vi "SavePodDataToFile.vi"(10 "Configuration Data":T1, 11 "Config file Refnum in":T2) -> (3 "Config file Refnum out":T2)   [LabVIEW 2014]
uses:
  <vilib>/Utility/config.llb/Config Data RefNum.ctl
  <vilib>/Utility/config.llb/Write Key (I32).vi
  <vilib>/Utility/config.llb/Write Key (String).vi
  <vilib>/Utility/config.llb/Write Key (Double).vi
  <vilib>/Utility/config.llb/Write Key (Boolean).vi
  <vilib>/Utility/config.llb/NI_LVConfig.lvlib
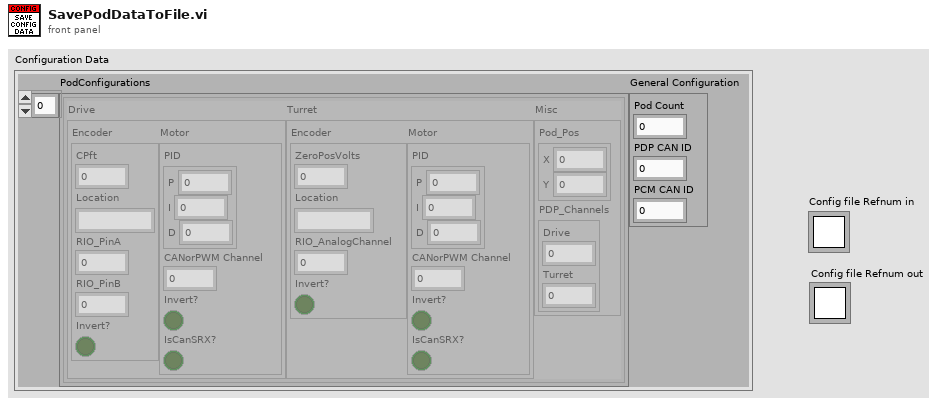
[diagram p1: front panel]
types:
  T1 = cluster{"PodConfigurations":cluster{"Drive":cluster{"Encoder":cluster{"CPft":dbl, "Location":string, "RIO_PinA":i32, "RIO_PinB":i32, "Invert?":bool}, "Motor":cluster{"PID":cluster{"P":dbl, "I":dbl, "D":dbl}, "CANorPWM Channel":i32, "Invert?":bool, "IsCanSRX?":bool}}, "Turret":cluster{"Encoder":cluster{"ZeroPosVolts":dbl, "Location":string, "RIO_AnalogChannel":i32, "Invert?":bool}, "Motor":cluster{"PID":cluster{"P":dbl, "I":dbl, "D":dbl}, "CANorPWM Channel":i32, "Invert?":bool, "IsCanSRX?":bool}}, "Misc":cluster{"Pod_Pos":cluster{"X":dbl, "Y":dbl}, "PDP_Channels":cluster{"Drive":i32, "Turret":i32}}}[], "General Configuration":cluster{"Pod Count":i32, "PDP CAN ID":i32, "PCM CAN ID":i32}}
  T2 = typedef "NI_LVConfig.lvlib/Config Data RefNum.ctl" = refnum<k1>
  T3 = cluster{"Drive":cluster{"Encoder":cluster{"CPft":dbl, "Location":string, "RIO_PinA":i32, "RIO_PinB":i32, "Invert?":bool}, "Motor":cluster{"PID":cluster{"P":dbl, "I":dbl, "D":dbl}, "CANorPWM Channel":i32, "Invert?":bool, "IsCanSRX?":bool}}, "Turret":cluster{"Encoder":cluster{"ZeroPosVolts":dbl, "Location":string, "RIO_AnalogChannel":i32, "Invert?":bool}, "Motor":cluster{"PID":cluster{"P":dbl, "I":dbl, "D":dbl}, "CANorPWM Channel":i32, "Invert?":bool, "IsCanSRX?":bool}}, "Misc":cluster{"Pod_Pos":cluster{"X":dbl, "Y":dbl}, "PDP_Channels":cluster{"Drive":i32, "Turret":i32}}}[]
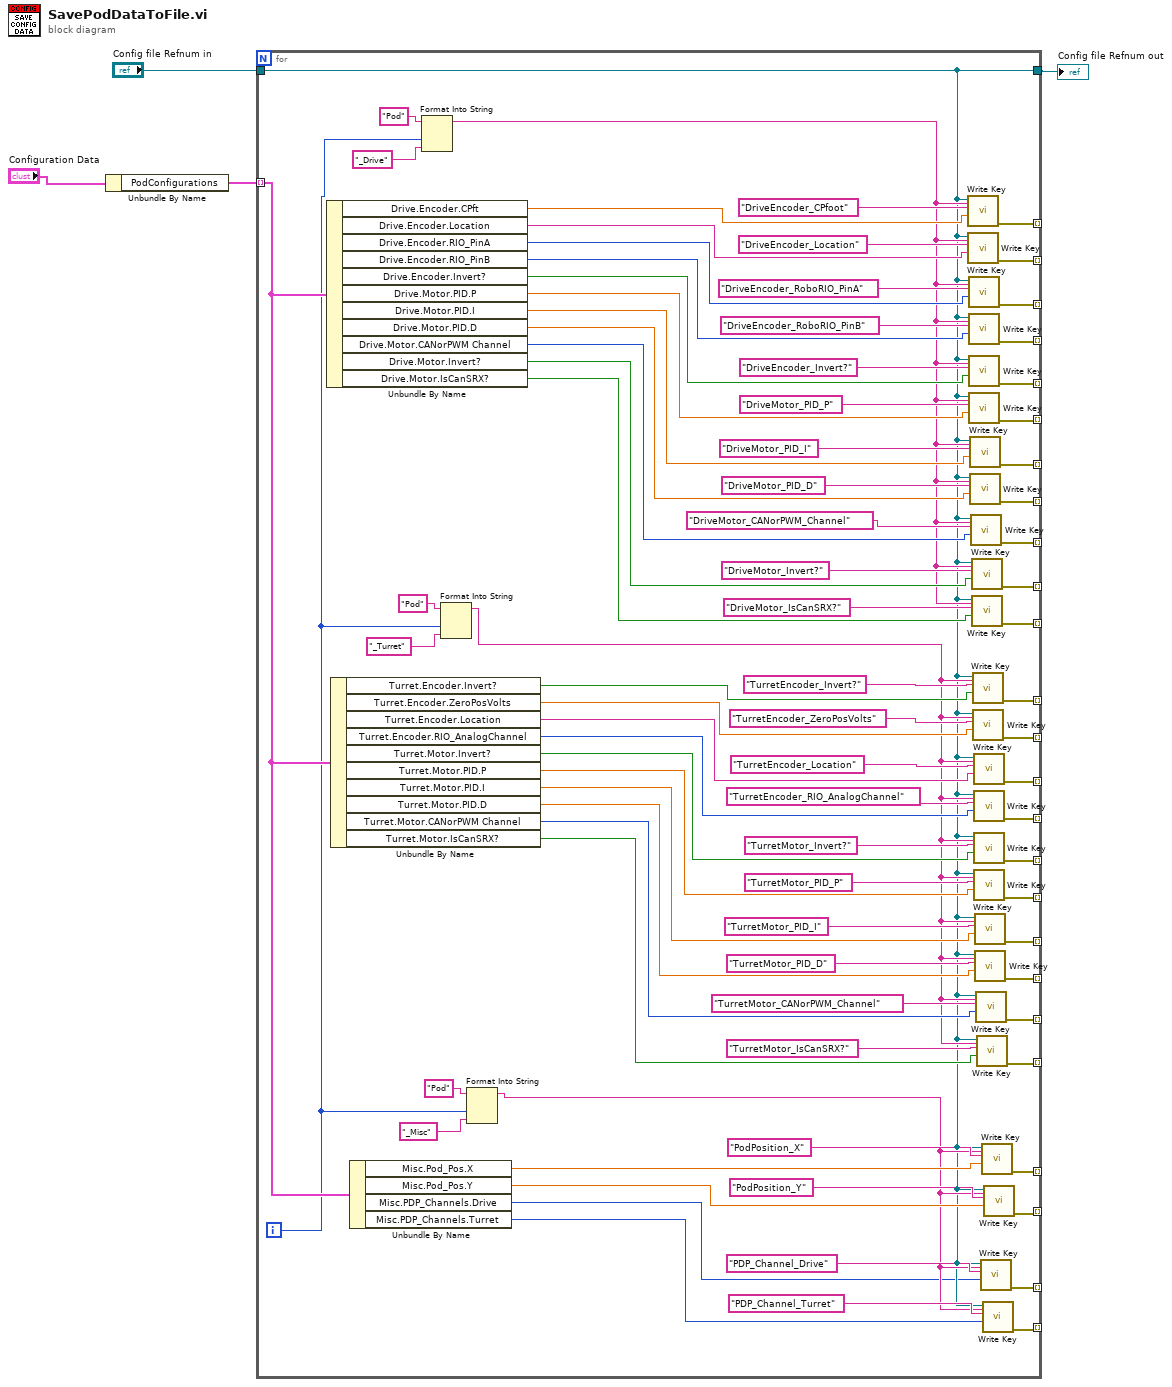
[diagram p0: block diagram]
diagram:
  n1 = Unbundle By Name("Configuration Data") -> ("PodConfigurations"=w4:T3)
  n2 = for {
    tunnel: "Config file Refnum in" -> [w7]
    tunnel: w4 -> [w43] mode=indexing
    tunnel: [w7] -> w2
    tunnel: [w37] -> _ mode=indexing
    tunnel: [w36] -> _ mode=indexing
    tunnel: [w35] -> _ mode=indexing
    tunnel: [w34] -> _ mode=indexing
    tunnel: [w33] -> _ mode=indexing
    tunnel: [w32] -> _ mode=indexing
    tunnel: [w31] -> _ mode=indexing
    tunnel: [w30] -> _ mode=indexing
    tunnel: [w29] -> _ mode=indexing
    tunnel: [w28] -> _ mode=indexing
    tunnel: [w27] -> _ mode=indexing
    tunnel: [w26] -> _ mode=indexing
    tunnel: [w25] -> _ mode=indexing
    tunnel: [w24] -> _ mode=indexing
    tunnel: [w23] -> _ mode=indexing
    tunnel: [w22] -> _ mode=indexing
    tunnel: [w21] -> _ mode=indexing
    tunnel: [w20] -> _ mode=indexing
    tunnel: [w19] -> _ mode=indexing
    tunnel: [w18] -> _ mode=indexing
    tunnel: [w17] -> _ mode=indexing
    tunnel: [w16] -> _ mode=indexing
    tunnel: [w15] -> _ mode=indexing
    tunnel: [w11] -> _ mode=indexing
    tunnel: [w12] -> _ mode=indexing
    i -> [w38]
    n3 = Unbundle By Name(w43) -> ("Drive.Encoder.CPft"=w88:dbl, "Drive.Encoder.Location"=w86:string, "Drive.Encoder.RIO_PinA"=w83:i32, "Drive.Encoder.RIO_PinB"=w82:i32, "Drive.Encoder.Invert?"=w77:bool, "Drive.Motor.PID.P"=w76:dbl, "Drive.Motor.PID.I"=w75:dbl, "Drive.Motor.PID.D"=w74:dbl, "Drive.Motor.CANorPWM Channel"=w70:i32, "Drive.Motor.Invert?"=w69:bool, "Drive.Motor.IsCanSRX?"=w68:bool)
    n4 = Unbundle By Name(w43) -> ("Turret.Encoder.Invert?"=w48:bool, "Turret.Encoder.ZeroPosVolts"=w50:dbl, "Turret.Encoder.Location"=w53:string, "Turret.Encoder.RIO_AnalogChannel"=w54:i32, "Turret.Motor.Invert?"=w59:bool, "Turret.Motor.PID.P"=w60:dbl, "Turret.Motor.PID.I"=w61:dbl, "Turret.Motor.PID.D"=w62:dbl, "Turret.Motor.CANorPWM Channel"=w65:i32, "Turret.Motor.IsCanSRX?"=w66:bool)
    n5 = Unbundle By Name(w43) -> ("Misc.Pod_Pos.X"=w14:dbl, "Misc.Pod_Pos.Y"=w13:dbl, "Misc.PDP_Channels.Drive"=w6:i32, "Misc.PDP_Channels.Turret"=w5:i32)
    n6 = Format Into String(initial string="Pod", w38, "_Drive") -> (resulting string=w67:string)  [unwired: 2 in, 1 out]
    n7 = Format Into String(initial string="Pod", w38, "_Turret") -> (resulting string=w44:string)  [unwired: 2 in, 1 out]
    n8 = Format Into String(initial string="Pod", w38, "_Misc") -> (resulting string=w8:string)  [unwired: 2 in, 1 out]
    n9 = call-poly <vilib>:"Write Key.vi"("section"=w67, "value"=w88, "key"="DriveEncoder_CPfoot", "refnum"=w7) -> ("error out"=w37:errorcluster)  [unwired: 5 in, 2 out]
    n10 = call-poly <vilib>:"Write Key.vi"("section"=w67, "value"=w86, "key"="DriveEncoder_Location", "refnum"=w7) -> ("error out"=w36:errorcluster)  [unwired: 5 in, 2 out]
    n11 = call-poly <vilib>:"Write Key.vi"("section"=w67, "value"=w83, "key"="DriveEncoder_RoboRIO_PinA", "refnum"=w7) -> ("error out"=w35:errorcluster)  [unwired: 5 in, 2 out]
    n12 = call-poly <vilib>:"Write Key.vi"("section"=w67, "value"=w82, "key"="DriveEncoder_RoboRIO_PinB", "refnum"=w7) -> ("error out"=w34:errorcluster)  [unwired: 5 in, 2 out]
    n13 = call-poly <vilib>:"Write Key.vi"("section"=w67, "value"=w77, "key"="DriveEncoder_Invert?", "refnum"=w7) -> ("error out"=w33:errorcluster)  [unwired: 5 in, 2 out]
    n14 = call-poly <vilib>:"Write Key.vi"("section"=w67, "value"=w76, "key"="DriveMotor_PID_P", "refnum"=w7) -> ("error out"=w32:errorcluster)  [unwired: 5 in, 2 out]
    n15 = call-poly <vilib>:"Write Key.vi"("section"=w67, "value"=w75, "key"="DriveMotor_PID_I", "refnum"=w7) -> ("error out"=w31:errorcluster)  [unwired: 5 in, 2 out]
    n16 = call-poly <vilib>:"Write Key.vi"("section"=w67, "value"=w74, "key"="DriveMotor_PID_D", "refnum"=w7) -> ("error out"=w30:errorcluster)  [unwired: 5 in, 2 out]
    n17 = call-poly <vilib>:"Write Key.vi"("section"=w67, "value"=w70, "key"="DriveMotor_CANorPWM_Channel", "refnum"=w7) -> ("error out"=w29:errorcluster)  [unwired: 5 in, 2 out]
    n18 = call-poly <vilib>:"Write Key.vi"("section"=w67, "value"=w69, "key"="DriveMotor_Invert?", "refnum"=w7) -> ("error out"=w28:errorcluster)  [unwired: 5 in, 2 out]
    n19 = call-poly <vilib>:"Write Key.vi"("section"=w67, "value"=w68, "key"="DriveMotor_IsCanSRX?", "refnum"=w7) -> ("error out"=w27:errorcluster)  [unwired: 5 in, 2 out]
    n20 = call-poly <vilib>:"Write Key.vi"("section"=w44, "value"=w48, "key"="TurretEncoder_Invert?", "refnum"=w7) -> ("error out"=w26:errorcluster)  [unwired: 5 in, 2 out]
    n21 = call-poly <vilib>:"Write Key.vi"("section"=w44, "value"=w50, "key"="TurretEncoder_ZeroPosVolts", "refnum"=w7) -> ("error out"=w25:errorcluster)  [unwired: 5 in, 2 out]
    n22 = call-poly <vilib>:"Write Key.vi"("section"=w44, "value"=w53, "key"="TurretEncoder_Location", "refnum"=w7) -> ("error out"=w24:errorcluster)  [unwired: 5 in, 2 out]
    n23 = call-poly <vilib>:"Write Key.vi"("section"=w44, "value"=w54, "key"="TurretEncoder_RIO_AnalogChannel", "refnum"=w7) -> ("error out"=w23:errorcluster)  [unwired: 5 in, 2 out]
    n24 = call-poly <vilib>:"Write Key.vi"("section"=w44, "value"=w59, "key"="TurretMotor_Invert?", "refnum"=w7) -> ("error out"=w22:errorcluster)  [unwired: 5 in, 2 out]
    n25 = call-poly <vilib>:"Write Key.vi"("section"=w44, "value"=w60, "key"="TurretMotor_PID_P", "refnum"=w7) -> ("error out"=w21:errorcluster)  [unwired: 5 in, 2 out]
    n26 = call-poly <vilib>:"Write Key.vi"("section"=w44, "value"=w61, "key"="TurretMotor_PID_I", "refnum"=w7) -> ("error out"=w20:errorcluster)  [unwired: 5 in, 2 out]
    n27 = call-poly <vilib>:"Write Key.vi"("section"=w44, "value"=w62, "key"="TurretMotor_PID_D", "refnum"=w7) -> ("error out"=w19:errorcluster)  [unwired: 5 in, 2 out]
    n28 = call-poly <vilib>:"Write Key.vi"("section"=w44, "value"=w65, "key"="TurretMotor_CANorPWM_Channel", "refnum"=w7) -> ("error out"=w18:errorcluster)  [unwired: 5 in, 2 out]
    n29 = call-poly <vilib>:"Write Key.vi"("section"=w44, "value"=w66, "key"="TurretMotor_IsCanSRX?", "refnum"=w7) -> ("error out"=w17:errorcluster)  [unwired: 5 in, 2 out]
    n30 = call-poly <vilib>:"Write Key.vi"("section"=w8, "value"=w6, "key"="PDP_Channel_Drive", "refnum"=w7) -> ("error out"=w11:errorcluster)  [unwired: 5 in, 2 out]
    n31 = call-poly <vilib>:"Write Key.vi"("section"=w8, "value"=w14, "key"="PodPosition_X", "refnum"=w7) -> ("error out"=w16:errorcluster)  [unwired: 5 in, 2 out]
    n32 = call-poly <vilib>:"Write Key.vi"("section"=w8, "value"=w5, "key"="PDP_Channel_Turret", "refnum"=w7) -> ("error out"=w12:errorcluster)  [unwired: 5 in, 2 out]
    n33 = call-poly <vilib>:"Write Key.vi"("section"=w8, "value"=w13, "key"="PodPosition_Y", "refnum"=w7) -> ("error out"=w15:errorcluster)  [unwired: 5 in, 2 out]
  }
  "Config file Refnum out" <- w2
